vi "Log Event.vi"(8 "error in (no error)":errorcluster, 10 "Event":T1, 11 "Logger in":refnum<class "Logger.lvclass">) -> (0 "error out":errorcluster, 3 "Logger out":refnum<class "Logger.lvclass">)   [LabVIEW 2019, in "Logger.lvlib" / "Logger.lvclass"]
uses:
  Logger.lvclass
  Sensors/Detector/Event.ctl
  Logger.lvclass/Logger.ctl
  Sensors/Detector/Muon Detector.lvclass
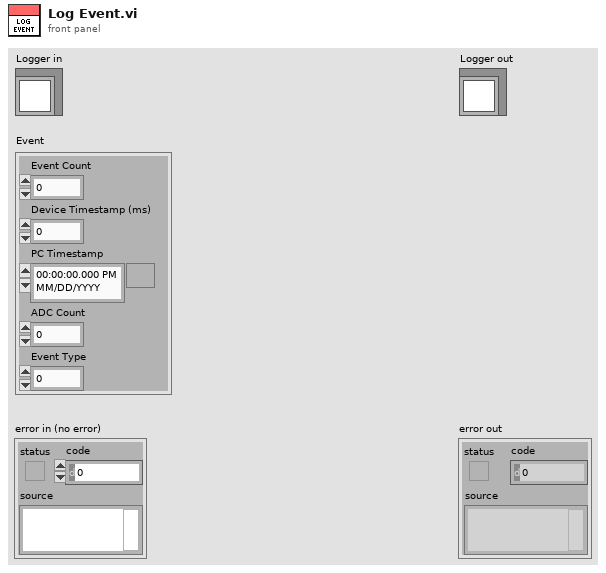
[diagram p1: front panel]
types:
  T1 = typedef "Muon Detector.lvclass/Event.ctl" = cluster{"Event Count":i32, "Device Timestamp (ms)":i32, "PC Timestamp":timestamp, "ADC Count":i32, "Event Type":u8}
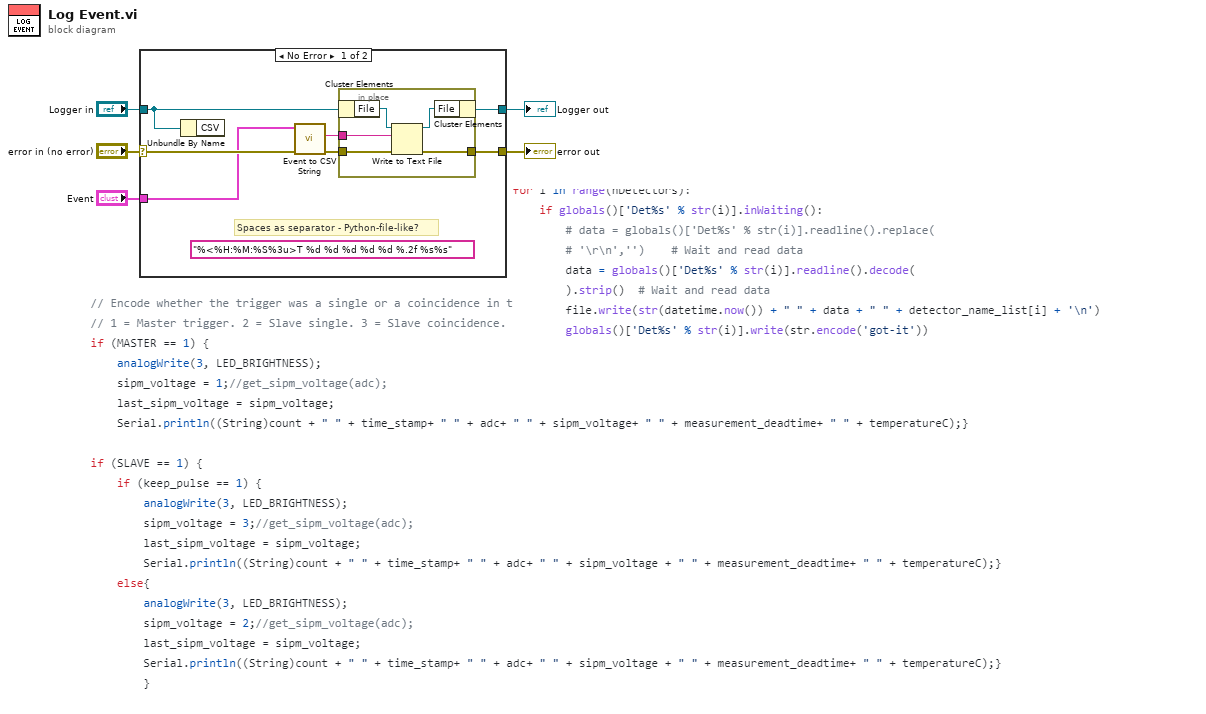
[diagram p0: block diagram]
diagram:
  n1 = case shown="No Error" "error in (no error)" {
    selector: "error in (no error)" -> [w9 w19]
    tunnel: [w10 w19] -> w4
    tunnel: [w12 w18] -> w2
    tunnel: "Logger in" -> [w8 w18]
    tunnel: "Event" -> [w7 _]
    frame No Error {
      (unwired) "%<%H:%M:%S%3u>T %d %d %d %d %d %.2f %s%s" ("format string")
      # "Spaces as separator - Python-file-like?"
      n2 = Unbundle By Name(w8) -> ()  [unwired: 1 out]
      n3 = call "Event to CSV String.vi"("error in (no error)"=w9, "Event"=w7) -> ("error out"=w11:errorcluster, "String"=w6:string)  [unwired: 8 in]
      n4 = in-place {
        in-place-border: w6 -> [w15]
        in-place-border: w11 -> [w14]
        in-place-border: [w13] -> w10
        n5 = in-place-cluster #1(w8) -> ("File"=w17:refnum<file>)
        n6 = Write to Text File(file (use dialog)=w17, text=w15, error in=w14) -> (refnum out=w16:refnum<file>, error out=w13:errorcluster)  [unwired: 1 in, 1 out]
        n7 = in-place-cluster #1("File"=w16) -> (w12:refnum<class "Logger.lvclass">)
      }
    }
    frame Error {
    }
  }
  "error out" <- w4
  "Logger out" <- w2
